vi "Send Email.vi"(6 "Message":string, 7 "Server Address":string, 8 "error in (no error)":errorcluster, 9 "Subject":string, 10 "Recipients":string, 11 "From":string) -> (0 "error out":errorcluster)   [LabVIEW 2020]
uses:
  <vilib>/smtpClient/Set Message Text.vi
  <vilib>/smtpClient/LabVIEWSMTPClient.lvlib
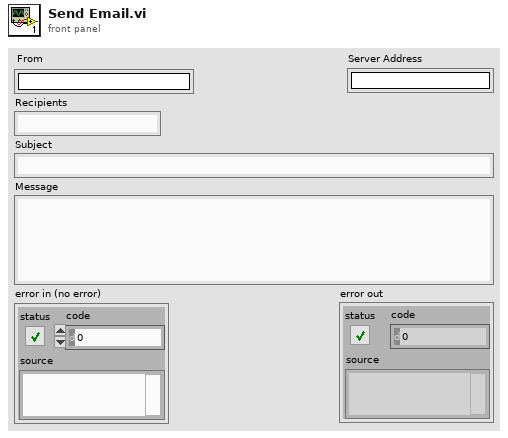
[diagram p1: front panel]
types:
  T1 = typedef "LabVIEWSMTPClient.lvlib/SmtpClientHandle.ctl" = refnum<k1>
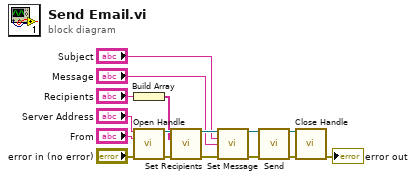
[diagram p0: block diagram]
diagram:
  n1 = Build Array("Recipients") -> (w10:string[])
  n2 = call <vilib>:"Open Handle.vi"("server address"="Server Address", "from"="From", "error in (no error)"="error in (no error)") -> ("handle out"=w12:T1, "error out"=w13:errorcluster)  [unwired: 11 in]
  n3 = call <vilib>:"Set Recipients.vi"("handle in"=w12, "to"=w10, "error in (no error)"=w13) -> ("handle out"=w9:T1, "error out"=w1:errorcluster)  [unwired: 11 in]
  n4 = call-poly <vilib>:"Set Message.vi"("handle in"=w9, "subject"="Subject", "plain text message"="Message", "error in (no error)"=w1) -> ("handle out"=w6:T1, "error out"=w3:errorcluster)  [unwired: 10 in]
  n5 = call <vilib>:"Send.vi"("handle in"=w6, "error in (no error)"=w3) -> ("handle out"=w5:T1, "error out"=w4:errorcluster)  [unwired: 11 in, 1 out]
  n6 = call <vilib>:"Close Handle.vi"("handle in"=w5, "error in (no error)"=w4) -> ("error out"=→"error out":errorcluster)  [unwired: 12 in, 1 out]
